vi "Kinect_init(SubVI).vi"(8 "error in (no error)":errorcluster, 11 "log_level":u32) -> (0 "error out":errorcluster, 3 "Context_handle":i64)   [LabVIEW 2017]
uses:
  libkinect_wrapper.dll
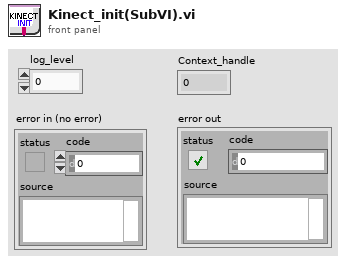
[diagram p1: front panel]
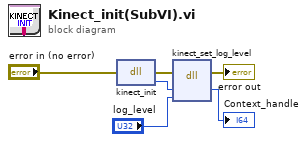
[diagram p0: block diagram]
diagram:
  n1 = dll-call lib="libkinect_wrapper.*" fn="kinect_init"(error in="error in (no error)") -> (error out=w2:errorcluster, "Context_handle"=w3:i64)  [unwired: 2 in, 1 out]
  n2 = dll-call lib="libkinect_wrapper.*" fn="kinect_set_log_level"(error in=w2, "Context_handle"=w3, "log_level"="log_level") -> (error out=→"error out":errorcluster, "Context_handle"=→"Context_handle":i64)  [unwired: 4 in, 1 out]
